vi "Write Value to Camera.vi"(8 "error in (no error)":errorcluster, 10 "Attribute Information":T1, 11 "Cam Attr IF in":refnum<class "Cam Attr IF.lvclass">) -> (0 "error out":errorcluster, 3 "Cam Attr IF out":refnum<class "Cam Attr IF.lvclass">)   [LabVIEW 2020, in "Cam Attr IF.lvclass"]
uses:
  Cam Attr IF.lvclass
  Camera Attribute Info.ctl
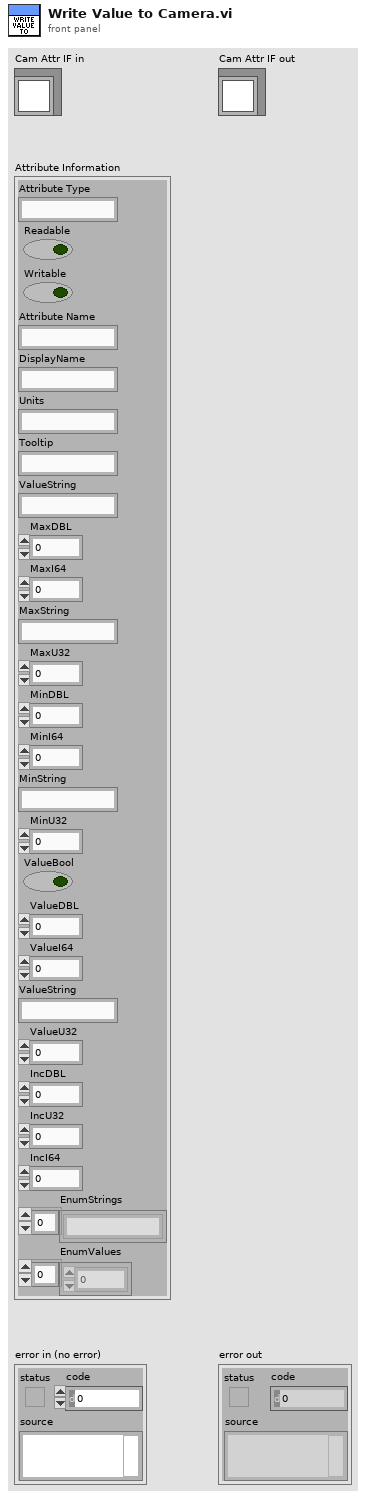
[diagram p1: front panel]
types:
  T1 = typedef "Camera Attribute Info.ctl" = cluster{"Attribute Type":string, "Readable":bool, "Writable":bool, "Attribute Name":string, "DisplayName":string, "Units":string, "Tooltip":string, "ValueString":string, "MaxDBL":dbl, "MaxI64":i64, "MaxString":string, "MaxU32":u32, "MinDBL":dbl, "MinI64":i64, "MinString":string, "MinU32":u32, "ValueBool":bool, "ValueDBL":dbl, "ValueI64 ":i64, "ValueString":string, "ValueU32":u32, "IncDBL":dbl, "IncU32":u32, "IncI64":i64, "EnumStrings":string[], "EnumValues":u32[]}
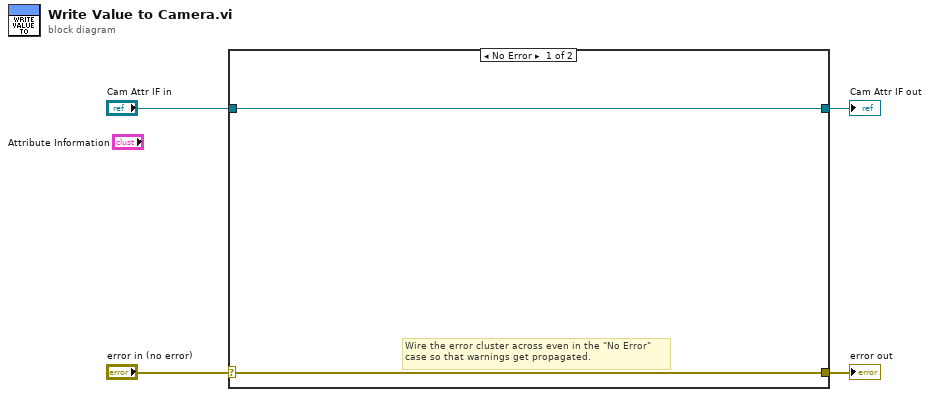
[diagram p0: block diagram]
diagram:
  n1 = case shown="No Error" "error in (no error)" {
    selector: "error in (no error)" -> [w5 w8]
    tunnel: [w5 w8] -> w3
    tunnel: [w6 w7] -> w1
    tunnel: "Cam Attr IF in" -> [w6 w7]
    frame No Error {
      # "Wire the error cluster across even in the \"No Error\"\ncase so that warnings get propagated."
    }
    frame Error {
    }
  }
  "error out" <- w3
  "Cam Attr IF out" <- w1
